vi "set gain.vi"(2 "error in (no error)":errorcluster, 3 "Gain":dbl=50.0, 4 "VISA resource name":refnum<visa-resource-name>="GPIB0::12::INSTR") -> (0 "error out":errorcluster, 1 "VISA resource name out":refnum<visa-resource-name>)   [LabVIEW 2017, in "MicrowaveAmplifier.lvlib"]
uses:
  MicrowaveAmplifier.lvlib
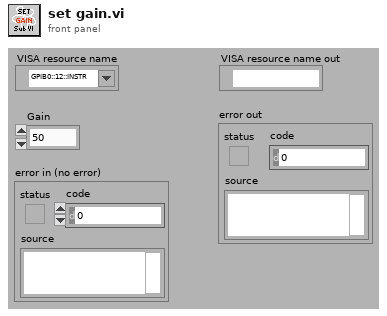
[diagram p1: front panel]
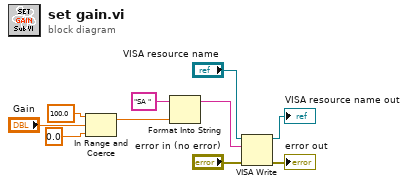
[diagram p0: block diagram]
diagram:
  n1 = In Range and Coerce(upper limit=100.0, x="Gain", lower limit=0.0) -> (coerced(x)=w8:dbl)  [unwired: 1 out]
  n2 = Format Into String(initial string="SA " ("write string"), w8) -> (resulting string=w10:string)  [unwired: 2 in, 1 out]
  n3 = VISA Write(VISA resource name="VISA resource name", write buffer=w10, error in (no error)="error in (no error)") -> (VISA resource name out=→"VISA resource name out":refnum<visa-resource-name>, error out=→"error out":errorcluster)  [unwired: 1 out]
